vi "Read 1 Screen Tap Position.vi"(8 "Error In":errorcluster, 11 "Leap Handle":T2) -> (0 "Error Out":errorcluster, 1 "Screen Tap Status":T1, 2 "Screen Tap Position":cluster{"X":sgl, "Y":sgl, "Z":sgl}, 3 "Leap Handle":T2)   [LabVIEW 2011, in "LMH-Leap.lvlib"]
doc: "Read one screen tap gesture position."
uses:
  LMH-Leap.lvlib
  Private/Type Defs/Leap Handle.ctl
  C:/github/makerhub/Leap/LabVIEW/vi.lib/MakerHub/Leap/Private/Libs/LeapCSharp.NET3.5.dll
  Private/Libs/LeapCSharp.NET3.5.dll
  Private/Type Defs/Gesture State.ctl
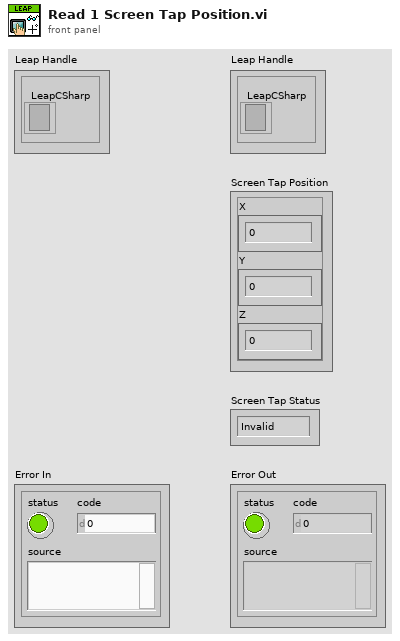
[diagram p1: front panel]
types:
  T1 = typedef "LMH-Leap.lvlib/Gesture State.ctl" = enum16{"Invalid", "Start", "Update", "Stop"}
  T2 = typedef "LMH-Leap.lvlib/Leap Handle.ctl" = cluster{"LeapCSharp":refnum<k24>}
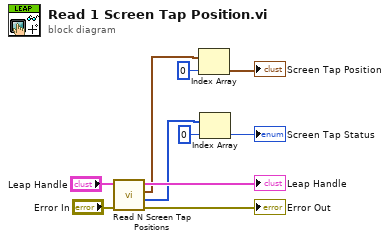
[diagram p0: block diagram]
diagram:
  n1 = call "Read N Screen Tap Positions.vi"("Error In"="Error In", "Leap Handle"="Leap Handle") -> ("Error Out"=→"Error Out":errorcluster, "Screen Tap Statuses"=w4:T1[], "Screen Tap Positions"=w3:cluster{"X":sgl, "Y":sgl, "Z":sgl}[], "Leap Handle"=→"Leap Handle":T2)  [unwired: 6 in]
  n2 = Index Array(array=w3, index=0) -> (element=→"Screen Tap Position":cluster{"X":sgl, "Y":sgl, "Z":sgl})
  n3 = Index Array(array=w4, index=0) -> (element=→"Screen Tap Status":T1)
